vi "change queue.vi"(10 "queue":refnum<class "identifying queue.lvclass">, 11 "communicator in":refnum<class "communicator.lvclass">) -> (3 "communicator out":refnum<class "communicator.lvclass">)   [LabVIEW 2015, in "communicator.lvclass"]
uses:
  communicator.lvclass
  communicator queue/identifying queue.lvclass
  communicator.lvclass/communicator.ctl
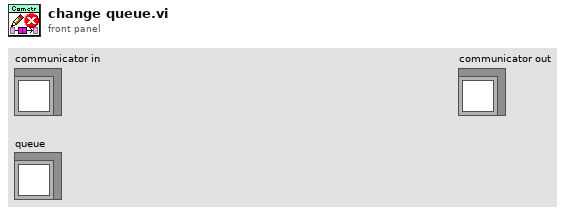
[diagram p1: front panel]
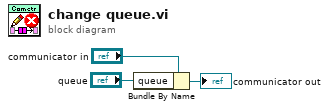
[diagram p0: block diagram]
diagram:
  n1 = Bundle By Name(cluster="communicator in", "queue"="queue") -> (→"communicator out":refnum<class "communicator.lvclass">)
